vi "Debug Log.vi"(9 "Write?":bool, 10 "Data":u8[](array[numeric]), 11 "Message":string) -> (2 "Transcript":string)   [LabVIEW 2015, in "Digikrom DK24x.lvlib"]
doc: "To enable logging:\n1. Right click on \"Project: Digikrom DK24x.lvproj\" in the Project Explorer window\n2. Select \"Conditional Disable Symbols\"\n3. Add a new symbol called DEBUG and set its value to TRUE"
uses:
  Digikrom DK24x.lvlib
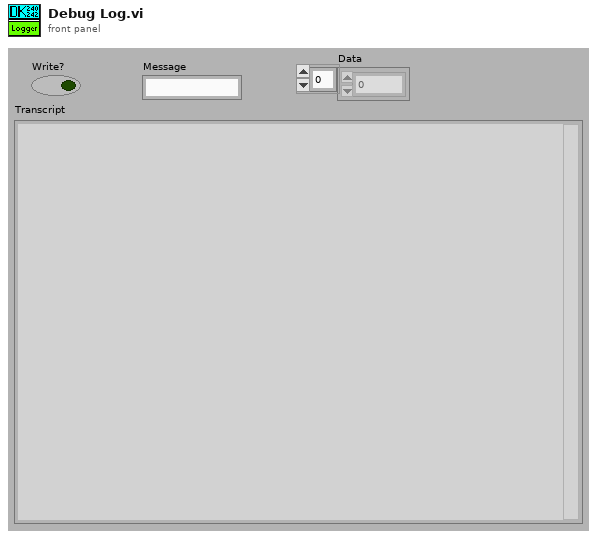
[diagram p1: front panel]
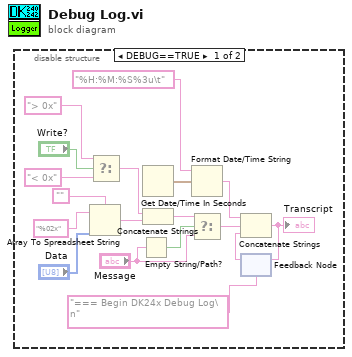
[diagram p0: block diagram]
diagram:
  n1 = disable-structure shown="DEBUG==TRUE" {
    frame condition #0 {
      n2 = Array To Spreadsheet String(delimiter (Tab)="", array="Data", 3:"%02x" ("format string")) -> (spreadsheet string=w5:string)
      n3 = Select(t="> 0x", s="Write?", f="< 0x") -> (s? t:f=w6:string)
      n4 = Empty String/Path?(string/path="Message") -> (empty?=w2:bool)
      n5 = Get Date/Time In Seconds() -> (seconds since 1Jan1904=w9:timestamp)
      n6 = Concatenate Strings(w6, w5) -> (w4:string)
      n7 = Format Date/Time String(time format string (%c)="%H:%M:%S%3u\t", seconds (now)=w9) -> (date/time string=w8:string)  [unwired: 1 out]
      n8 = Select(t=w4, s=w2, f="Message") -> (s? t:f=w1:string)
      n9 = feedback #1("=== Begin DK24x Debug Log\n") -> (w11:string)
      n10 = Concatenate Strings(w8, w1, w11) -> (w18:string)
      "Transcript" <- w18
      n11 = feedback-in #1(w18) -> ()
    }
    frame condition #1 (active) {
    }
  }
